vi "Create Directory Array.vi"(9 "Relative Path":string="models/in/nested/folder", 10 "Root Folder":string="/home/lvuser") -> (1 "Directory Array":string[](array[string]))   [LabVIEW 2020]
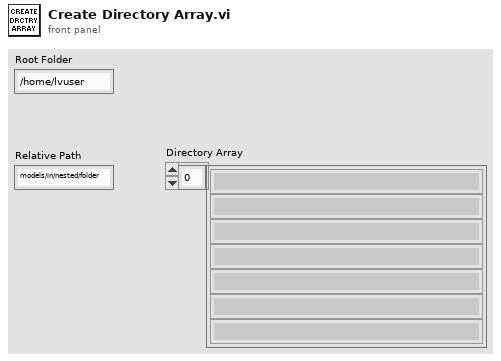
[diagram p1: front panel]
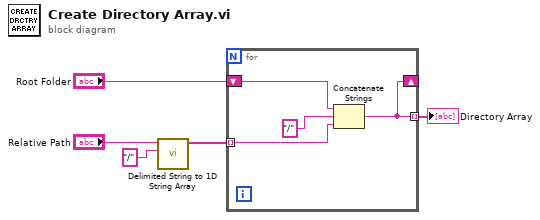
[diagram p0: block diagram]
diagram:
  n1 = call <vilib>:"Delimited String to 1D String Array.vi"("delimiter"="/", "delimited string"="Relative Path") -> ("string array"=w2:string[])  [unwired: 9 in]
  n2 = for {
    tunnel: w2 -> [w7] mode=indexing
    shift-right: [w6] -> _
    shift-left: "Root Folder" -> [w9]
    tunnel: [w6] -> w1 mode=indexing
    n3 = Concatenate Strings(w9, "/" ("delimiter"), w7) -> (w6:string)
  }
  "Directory Array" <- w1
